vi "MoveForward.vi"(4 "Loop Wait Delay":i32, 5 "Range":cluster{"output high":dbl, "output low":dbl}={"output high"=1.0, "output low"=-0.4} {"output low" format="%.2f"; "output high" format="%.2f"}, 6 "Delay After":i32, 7 "Gains":T1={"proportional gain (Kc)"=1.0, "integral time (Ti, min)"=0.01, "derivative time (Td, min)"=0.0} {"derivative time (Td, min)" format="%.3f"; "integral time (Ti, min)" format="%.3f"; "proportional gain (Kc)" format="%.3f"}, 8 "Reset":bool, 9 "Precision":dbl=0.5 format="%#_13g", 10 "Encoder Count":dbl, 11 "Distance":dbl) -> (2 "Output":dbl, 3 "Finished?":bool)   [LabVIEW 2019]
panel:
  out "PID":cluster{"Distance":dbl, "Encoder Count":dbl}(graph)
  out "Is Ramp On?":bool
  in  "Limiter":dbl=1.0
  in  "Integral Range":dbl=10000.0
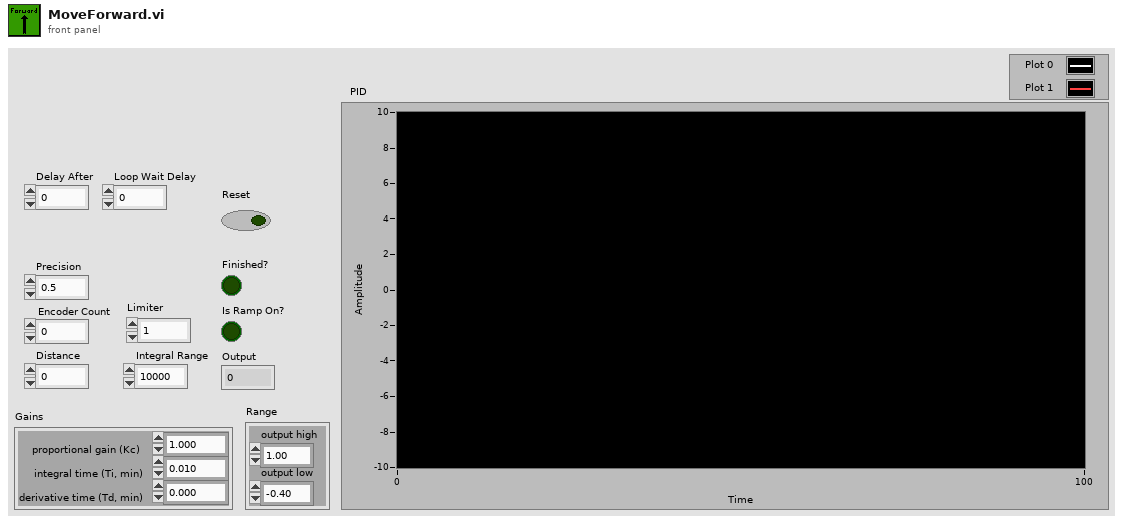
[diagram p1: front panel]
types:
  T1 = cluster{"proportional gain (Kc)":dbl, "integral time (Ti, min)":dbl, "derivative time (Td, min)":dbl}
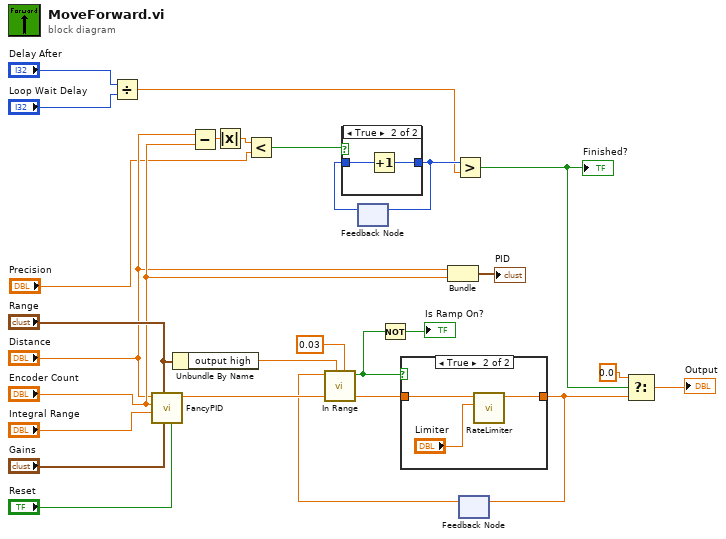
[diagram p0: block diagram]
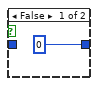
[diagram p2: hidden frame]
diagram:
  n1 = Divide(x="Delay After", y="Loop Wait Delay") -> (x/y=w3:dbl)
  n2 = call "FancyPID.vi"("Reset"="Reset", "Gains"="Gains", "Range"="Range", "Integral Range"="Integral Range", "Process variable"="Encoder Count", "Setpoint"="Distance") -> ("output"=w24:dbl)  [unwired: 5 in]
  n3 = Unbundle By Name("Range") -> ("output high"=w20:dbl)
  n4 = Subtract(x="Distance", y="Encoder Count") -> (x-y=w11:dbl)
  n5 = Absolute Value(x=w11) -> (abs(x)=w10:dbl)
  n6 = Less?(x=w10, y="Precision") -> (x < y?=w6:bool)
  n7 = feedback #1() -> (w7:i32)  [unwired: 1 in]
  n8 = case shown="True" w6 {
    tunnel: [0 w29] -> w8
    tunnel: w7 -> [_ w28]
    frame False {
    }
    frame True {
      n9 = Increment(x=w28) -> (x+1=w29:i32)
    }
  }
  n10 = feedback-in #1(w8) -> ()
  n11 = Bundle("Distance"="Distance", "Encoder Count"="Encoder Count") -> (→"PID":cluster{"Distance":dbl, "Encoder Count":dbl})  [unwired: 1 in]
  n12 = Greater?(x=w8, y=w3) -> (0:w2:bool)
  "Finished?" <- w2
  n13 = feedback #2() -> (w17:dbl)  [unwired: 1 in]
  n14 = call "In Range.vi"("Range"=0.03, "Setpoint"=w20, "Value"=w17) -> ("in range?"=w16:bool)  [unwired: 8 in]
  n15 = Not(x=w16) -> (.not. x?=→"Is Ramp On?":bool)
  n16 = case shown="True" w16 {
    tunnel: w24 -> [w30 w33]
    tunnel: [w30 w31] -> w18
    frame False {
    }
    frame True {
      n17 = call "RateLimiter.vi"("Max dx/dt"="Limiter", "Input"=w33) -> ("Output"=w31:dbl)  [unwired: 9 in]
    }
  }
  n18 = feedback-in #2(w18) -> ()
  n19 = Select(t=0.0, s=w2, f=w18) -> (s? t:f=→"Output":dbl)
